vi "Get 2D Pixel Array.vi"(11 "image data":T1) -> (3 "2D Pixel Array":u32[][](array[numeric]))   [LabVIEW 2015, in "Image Comparison.lvclass"]
uses:
  Image Comparison.lvclass
  <vilib>/picture/picture.llb/imagedata.ctl
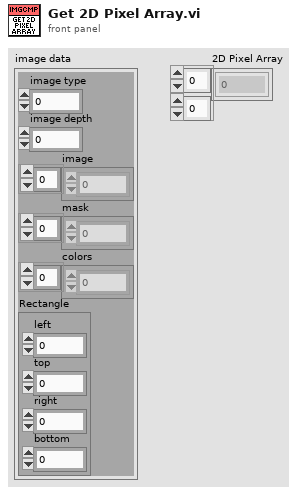
[diagram p1: front panel]
types:
  T1 = typedef "imagedata.ctl" = cluster{"image type":i32, "image depth":i32, "image":u8[], "mask":u8[], "colors":u32[], "Rectangle":cluster{"left":i16, "top":i16, "right":i16, "bottom":i16}}
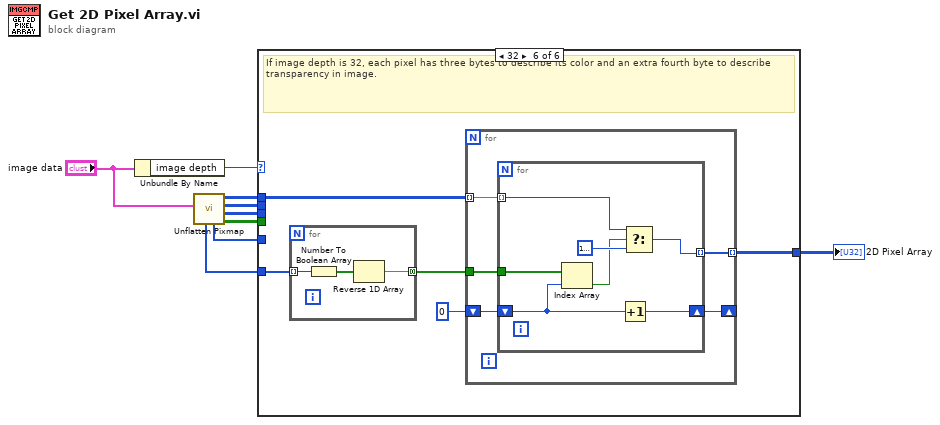
[diagram p0: block diagram]
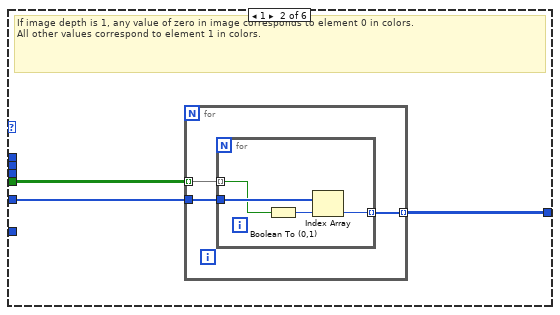
[diagram p3: hidden frame]
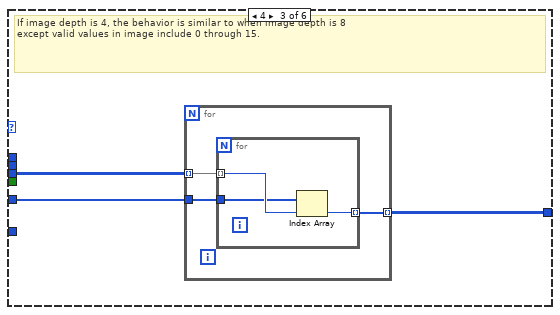
[diagram p4: hidden frame]
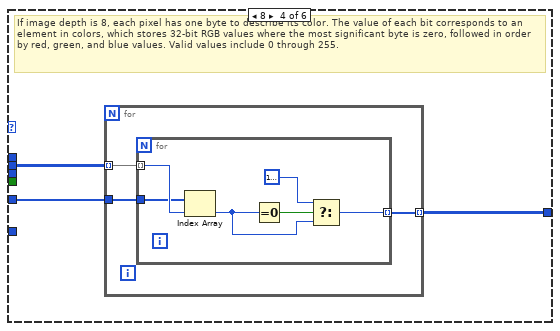
[diagram p5: hidden frame]
diagram:
  n1 = Unbundle By Name("image data") -> ("image depth"=w9:i32)
  n2 = call <vilib>:"Unflatten Pixmap.vi"("image data"="image data") -> ("1-bit pixmap"=w4:bool[][], "4-bit pixmap"=w5:u8[][], "8-bit pixmap"=w7:u8[][], "24-bit pixmap"=w3:u32[][], "colors"=w6:u32[], "mask"=w1:u8[])  [unwired: 4 in, 1 out]
  n3 = case shown="32" w9 {
    tunnel: [_ w10 w20 w29 w41 w42] -> w2
    tunnel: w7 -> [_ _ _ w31 _ _]
    tunnel: w6 -> [_ w12 w22 w30 _ _]
    tunnel: w5 -> [_ _ w21 _ _ _]
    tunnel: w4 -> [_ w11 _ _ _ _]
    tunnel: w3 -> [_ _ _ _ w41 w44]
    tunnel: w1 -> [_ _ _ _ _ w46]
    frame Default {
      # "Unused"
    }
    frame 1 {
      # "If image depth is 1, any value of zero in image corresponds to element 0 in colors. \nAll other values correspond to element 1 in colors."
      n4 = for {
        tunnel: [w15] -> w10 mode=indexing
        tunnel: w12 -> [w14]
        tunnel: w11 -> [w13] mode=indexing
        n5 = for {
          tunnel: w14 -> [w19]
          tunnel: [w18] -> w15 mode=indexing
          tunnel: w13 -> [w17] mode=indexing
          n6 = Boolean To (0,1)(Boolean=w17) -> (0, 1=w16:i16)
          n7 = Index Array(array=w19, index=w16) -> (element=w18:u32)
        }
      }
    }
    frame 4 {
      # "If image depth is 4, the behavior is similar to when image depth is 8 \nexcept valid values in image include 0 through 15."
      n8 = for {
        tunnel: [w25] -> w20 mode=indexing
        tunnel: w21 -> [w24] mode=indexing
        tunnel: w22 -> [w23]
        n9 = for {
          tunnel: [w27] -> w25 mode=indexing
          tunnel: w24 -> [w28] mode=indexing
          tunnel: w23 -> [w26]
          n10 = Index Array(array=w26, index=w28) -> (element=w27:u32)
        }
      }
    }
    frame 8 {
      # "If image depth is 8, each pixel has one byte to describe its color. The value of each bit corresponds to an element in colors, which stores 32-bit RGB values where the most significant byte is zero, followed in order by red, green, and blue values. Valid values include 0 through 255."
      n11 = for {
        tunnel: [w34] -> w29 mode=indexing
        tunnel: w31 -> [w33] mode=indexing
        tunnel: w30 -> [w32]
        n12 = for {
          tunnel: [w35] -> w34 mode=indexing
          tunnel: w33 -> [w40] mode=indexing
          tunnel: w32 -> [w39]
          n13 = Index Array(array=w39, index=w40) -> (element=w37:u32)
          n14 = Equal To 0?(x=w37) -> (x = 0?=w38:bool)
          n15 = Select(t=u32 16777216, s=w38, f=w37) -> (s? t:f=w35:u32)
        }
      }
    }
    frame 24 {
      # "If image depth is 24, each pixel has three bytes to describe its color in image. When the image depth is 24, the behavior is similar to when image depth is 32. However, 24-bit images do not have an extra fourth byte to describe transparency."
    }
    frame 32 {
      # "If image depth is 32, each pixel has three bytes to describe its color and an extra fourth byte to describe transparency in image."
      n16 = for {
        tunnel: w46 -> [w61] mode=indexing
        tunnel: [w59] -> w45 mode=concatenating
        n17 = Number To Boolean Array(number=w61) -> (Boolean array=w60:bool[])
        n18 = Reverse 1D Array(array=w60) -> (reversed array=w59:bool[])
      }
      n19 = for {
        tunnel: w45 -> [w51]
        tunnel: w44 -> [w50] mode=indexing
        shift-right: [w48] -> _
        shift-left: 0 -> [w49]
        tunnel: [w47] -> w42 mode=indexing
        n20 = for {
          tunnel: w50 -> [w58] mode=indexing
          tunnel: w51 -> [w55]
          tunnel: [w56] -> w47 mode=indexing
          shift-right: [w53] -> w48
          shift-left: w49 -> [w54]
          n21 = Index Array(array=w55, index=w54) -> (element=w52:bool)
          n22 = Increment(x=w54) -> (x+1=w53:i32)
          n23 = Select(t=w58, s=w52, f=u32 16777216) -> (s? t:f=w56:u32)
        }
      }
    }
  }
  "2D Pixel Array" <- w2
